vi "Configure Single Step Mode.vi"(0 "VISA resource name":refnum<visa-resource-name>, 5 "Single Step Mode (F:Disable)":bool, 11 "error in (no error)":errorcluster) -> (4 "VISA resource name out":refnum<visa-resource-name>, 15 "error out":errorcluster)   [LabVIEW 2020, in "eec 6700.lvlib"]
doc: "Sets the <B>Single Step Mode</B> in the power source instrument.\n\nNote : supported in Program mode only.\n\nThe single step parameter controls how the instrument will proceed from one test step to the next in a testing sequence when in the Auto Run mode of program. \n\nWhen the parameter is selected on the source will sequence from one test step to the next only when the test/reset key is press between each step. When the single step parameter is on the source will pause after each step has completed a test routine and passed based on the programmed testing parameters. If a pass occurs for the step the operator can proceed to the next step in the sequence. If a failure occurs for the step the operator will not be able to proceed in the test sequence. They will have to restart from the beginning of the test sequence or step number one.\n\nIf the parameter is selected off the source will automatically sequence from one step the next regardless if a pass or failure has occurred for a particular step."
uses:
  <instrlib>/eec 6700/eec 6700.lvlib
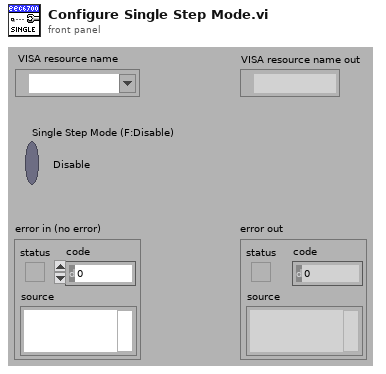
[diagram p1: front panel]
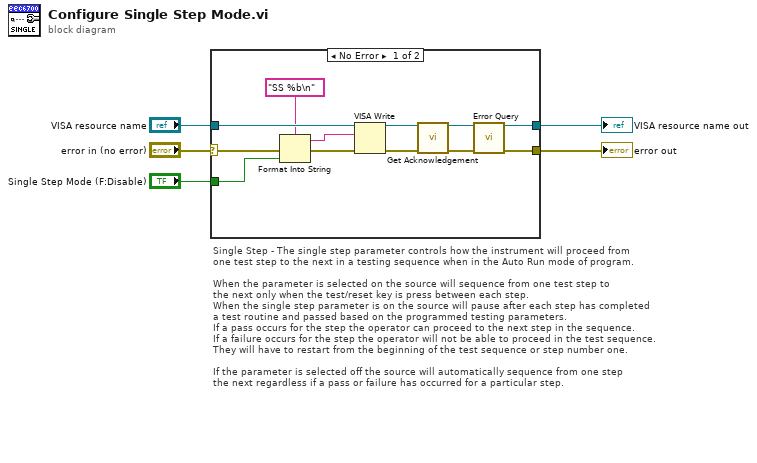
[diagram p0: block diagram]
diagram:
  # "Single Step - The single step parameter controls how the instrument will proceed from \none test step to the next in a testing sequence when in the Auto Run mode of program.  \n\nWhen the parameter is selected on the source will sequence from one test step to \nthe next only when the test/reset key is press between each step.  \nWhen the single step parameter is on the source will pause after each step has completed\na test routine and passed based on the programmed testing parameters.  \nIf a pass occurs for the step the operator can proceed to the next step in the sequence.  \nIf a failure occurs for the step the operator will not be able to proceed in the test sequence.  \nThey will have to restart from the beginning of the test sequence or step number one.\n\nIf the parameter is selected off the source will automatically sequence from one step \nthe next regardless if a pass or failure has occurred for a particular step."
  n1 = case shown="No Error" "error in (no error)" {
    selector: "error in (no error)" -> [w12 w19]
    tunnel: "VISA resource name" -> [w17 w18]
    tunnel: [w14 w18] -> w4
    tunnel: [w13 w19] -> w3
    tunnel: "Single Step Mode (F:Disable)" -> [w10 _]
    frame No Error {
      n2 = Format Into String(format string="SS %b\n" ("Command"), error in=w12, w10) -> (resulting string=w16:string, error out=w11:errorcluster)  [unwired: 1 in]
      n3 = VISA Write(VISA resource name=w17, write buffer=w16, error in (no error)=w11) -> (VISA resource name out=w7:refnum<visa-resource-name>, error out=w6:errorcluster)  [unwired: 1 out]
      n4 = call <instrlib>:"Get Acknowledgement.vi"("VISA resource name"=w7, "error in (no error)"=w6) -> ("VISA resource name out"=w8:refnum<visa-resource-name>, "error out"=w9:errorcluster)  [unwired: 12 in]
      n5 = call <instrlib>:"Error Query.vi"("VISA resource name"=w8, "error in (no error)"=w9) -> ("VISA resource name out"=w14:refnum<visa-resource-name>, "error out"=w13:errorcluster)  [unwired: 10 in, 2 out]
    }
    frame Error {
    }
  }
  "error out" <- w3
  "VISA resource name out" <- w4
